vi "SubVI2.vi"() -> (3 "Gauge":dbl)   [LabVIEW 2018]
panel:
  in  "OK Button":bool
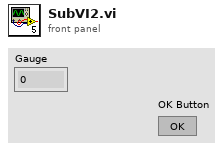
[diagram p1: front panel]
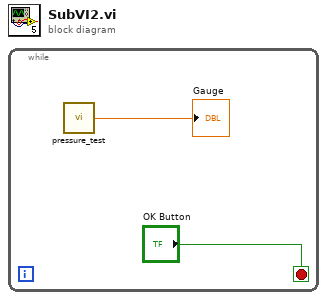
[diagram p0: block diagram]
diagram:
  n1 = while {
    stop <- "OK Button" stop-if-true
    n2 = call "pressure_test.vi"() -> ("Gauge"=→"Gauge":dbl)  [unwired: 1 in]
  }
